vi "Math-Uniform Random Number (I32, 1D).vi"(3 "Replace?":bool, 4 "N":i32, 5 "Ymin":i32, 6 "Ymax":i32) -> (1 "Random Ints":i32[](array[numeric]))   [LabVIEW 2020]
uses:
  LinSpace (start-stop-step).vi
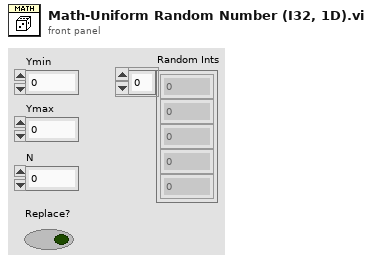
[diagram p1: front panel]
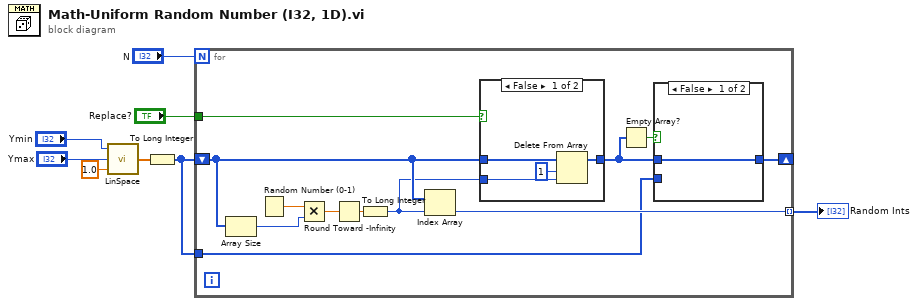
[diagram p0: block diagram]
diagram:
  n1 = call-poly "LinSpace.vi"("Step"=1.0, "Stop"="Ymax", "Start"="Ymin") -> ("Array"=w6:dbl[])  [unwired: 1 in, 1 out]
  n2 = To Long Integer(number=w6) -> (32bit integer=w1:i32[])
  n3 = for {
    N: "N" -> [_]
    shift-right: [w10] -> _
    shift-left: w1 -> [w15]
    tunnel: [w14] -> w3 mode=indexing
    tunnel: "Replace?" -> [w16]
    tunnel: w1 -> [w9]
    n4 = Array Size(array=w15) -> (size(s)=w17:i32)
    n5 = Random Number (0-1)() -> (number: 0 to 1=w20:dbl)
    n6 = Multiply(x=w20, y=w17) -> (x*y=w19:dbl)
    n7 = Round Toward -Infinity(1:w19) -> (0:w18:dbl)
    n8 = To Long Integer(number=w18) -> (32bit integer=w13:i32)
    n9 = Index Array(array=w15, index=w13) -> (element=w14:i32)
    n10 = case shown="False" w16 {
      tunnel: w15 -> [w26 w27]
      tunnel: [w25 w27] -> w11
      tunnel: w13 -> [w24 _]
      frame False {
        n11 = Delete From Array(array=w26, length=1, index=w24) -> (array with subset deleted=w25:i32[])  [unwired: 1 out]
      }
      frame True {
      }
    }
    n12 = Empty Array?(array=w11) -> (empty?=w12:bool)
    n13 = case shown="False" w12 {
      tunnel: w11 -> [w21 _]
      tunnel: [w21 w22] -> w10
      tunnel: w9 -> [_ w22]
      frame False {
      }
      frame True {
      }
    }
  }
  "Random Ints" <- w3
